vi "Concatenate Sequences.vi"(8 "error in (no error)":errorcluster, 11 "Scheduler in":refnum<class "Scheduler.lvclass">=refnum) -> (0 "error out":errorcluster, 3 "Scheduler out":refnum<class "Scheduler.lvclass">)   [LabVIEW 2020, in "CIRCUS_uServices.lvlib" / "Holy Trinity.lvlib" / "Scheduler.lvlib" / "Scheduler.lvclass"]
uses:
  Scheduler.lvclass
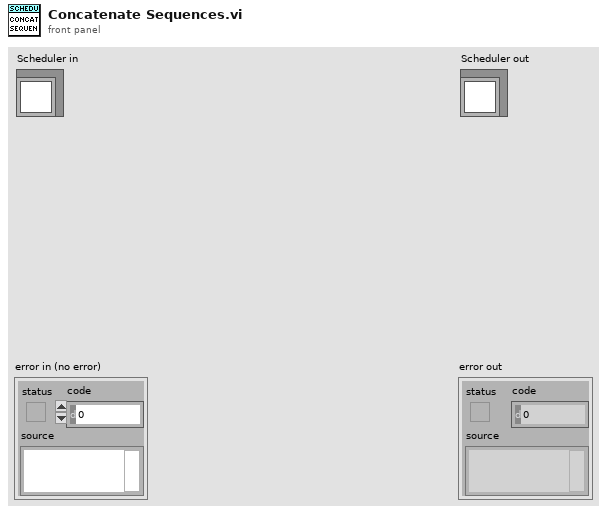
[diagram p1: front panel]
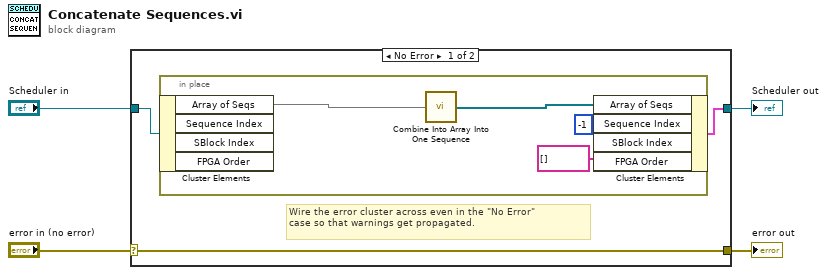
[diagram p0: block diagram]
diagram:
  n1 = case shown="No Error" "error in (no error)" {
    selector: "error in (no error)" -> [w7 w13]
    tunnel: [w7 w13] -> w3
    tunnel: [w5 w12] -> w1
    tunnel: "Scheduler in" -> [w6 w12]
    frame No Error {
      # "Wire the error cluster across even in the \"No Error\"\ncase so that warnings get propagated."
      n2 = in-place {
        w10 = -1 ("Sequence Index")
        n3 = in-place-cluster #1(w6) -> ("Array of Seqs"=w8)  [unwired: 3 out]
        n4 = call "Combine Into Array Into One Sequence.vi"("Array of Seqs in"=w8) -> ("Array of Seqs out"=w11:refnum<class "Sequence of SBlocks.lvclass">[])
        n5 = in-place-cluster #1("Array of Seqs"=w11, "Sequence Index"=w10, "SBlock Index"=w10, "FPGA Order"=string[] [] ("Kasli Order")) -> (w5:cluster{})
      }
    }
    frame Error {
    }
  }
  "error out" <- w3
  "Scheduler out" <- w1
